vi "Database-Changeover.vi"(8 "error in":errorcluster, 10 "PLCchangeover":T2, 11 "Idx":i32) -> (0 "error out":errorcluster, 2 "PCchangeover":T1 {"TVH" format="%.3f"; "TVL" format="%.3f"; "TP" format="%.3f"})   [LabVIEW 2016]
doc: "Go to DB->WriteStationValues action\nReturn boolean flag to show if data was saved to DB successfully\n\nWabco 2017 All right reserved\nAuthor: maciej.szupienko@wabco-auto.com"
uses:
  Database.Action.ctl
  Drivers/PLC/LowLevel/PLC.DataBlock.PCchangeover.ctl
  Drivers/PLC/LowLevel/PLC.DataBlock.PLCchangeover.ctl
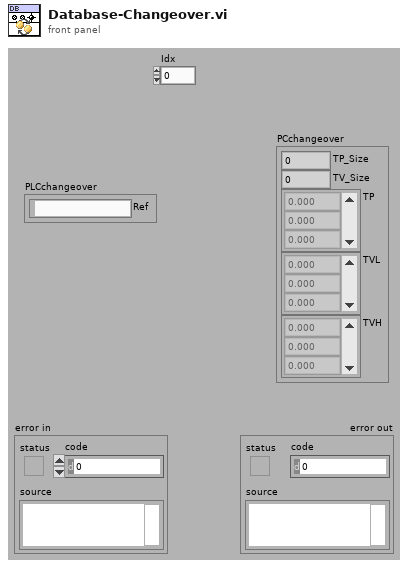
[diagram p1: front panel]
types:
  T1 = typedef "PLC.DataBlock.PCchangeover.ctl" = cluster{"TP_Size":u8, "TV_Size":u8, "TP":sgl[], "TVL":sgl[], "TVH":sgl[]}
  T2 = typedef "PLC.DataBlock.PLCchangeover.ctl" = cluster{"Ref":string}
  T3 = typedef "Database.Action.ctl" = enum32{"idle", "constructor", "destructor", "--- DB ---", "Setup", "Disconnect", "Connect", "GetAllStatuses"}
  T4 = typedef "Database.Data.Status.ctl" = cluster{"Run":bool, "Handle":i32, "ConnTS":timestamp, "DbTime":timestamp, "DbTimeOffset":dbl, "LastVariant":string, "LastSerial":string, "LastDataTS":timestamp, "LastStatus":i32}
  T5 = typedef "Cache.TestSteps.Fglb.TestData.ctl" = cluster{"Ref":string, "Desc":string, "P":T6, "PS":T7, "PP":T8[], "TS":cluster{"TS":T9, "TV":T10[], "TP":T11[]}[], "Units":T12[]}
  T6 = typedef "ProdaNG.Process.ctl" = cluster{"i_id":i32, "productionLineId":i32, "releaseId":i32, "contentId":string, "previewId":string, "mdReason":string, "mdUser":string, "mdTime":string, "description":string}
  T7 = typedef "ProdaNG.ProcessStep.ctl" = cluster{"i_id":i32, "processId":i32, "systemId":i32, "releaseId":i32, "processSequence":i32, "limitYellow":dbl, "limitRed":dbl, "mdReason":string, "mdUser":string, "mdTime":string, "filename":string, "transfer":string, "description":string}
  T8 = typedef "ProdaNG.ProcessStepParam.ctl" = cluster{"i_id":i32, "processStepId":i32, "unitId":i32, "contentId":string, "previewId":string, "value":dbl, "valueText":string, "paramSequence":i32, "history":i32, "mdReason":string, "mdUser":string, "mdTime":string, "description":string}
  T9 = typedef "ProdaNG.TestStep.ctl" = cluster{"i_id":i32, "processStepId":i32, "testSequence":i32, "testOrder":i32, "mdReason":string, "mdUser":string, "mdTime":string, "description":string}
  T10 = typedef "ProdaNG.TestValue.ctl" = cluster{"i_id":i32, "testStepId":i32, "releaseId":i32, "unitId":i32, "contentId":string, "previewId":string, "maximum":dbl, "minimum":dbl, "valueText":string, "testValueSequence":i32, "history":i32, "mdReason":string, "mdUser":string, "mdTime":string, "description":string}
  T11 = typedef "ProdaNG.TestStepParam.ctl" = cluster{"i_id":i32, "testStepId":i32, "unitId":i32, "contentId":string, "previewId":string, "value":dbl, "valueText":string, "paramSequence":i32, "history":i32, "mdReason":string, "mdUser":string, "mdTime":string, "description":string}
  T12 = typedef "ProdaNG.Unit.ctl" = cluster{"i_id":i32, "name":string, "mdReason":string, "mdUser":string, "mdTime":string, "description":string}
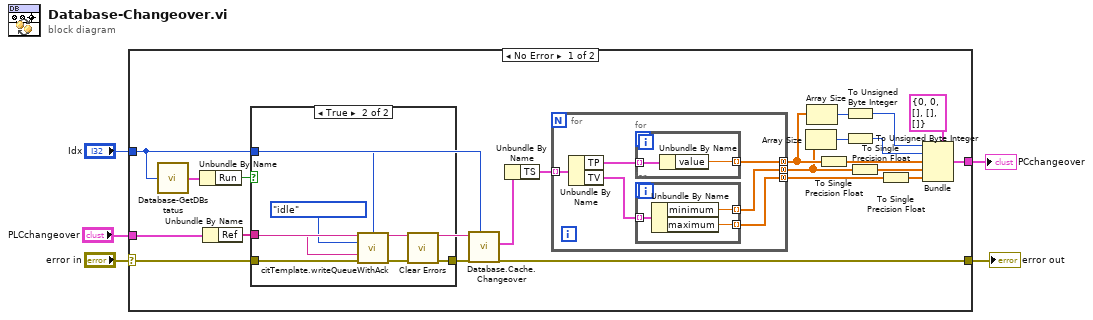
[diagram p0: block diagram]
diagram:
  n1 = case shown="No Error" "error in" {
    selector: "error in" -> [w27 w46]
    tunnel: [w24 w46] -> w4
    tunnel: "Idx" -> [w22 _]
    tunnel: "PLCchangeover" -> [w7 _]
    tunnel: [w11 _] -> w1
    frame No Error {
      n2 = call "Database-GetDBstatus.vi"("Idx"=w22) -> ("Status"=w26:T4)
      n3 = Unbundle By Name(w26) -> ("Run"=w25:bool)
      n4 = Unbundle By Name(w7) -> ("Ref"=w6:string)
      n5 = case shown="True" w25 {
        tunnel: w27 -> [w39 w45]
        tunnel: [w39 w42] -> w23
        tunnel: w22 -> [_ w44]
        tunnel: w6 -> [_ w41]
        frame False {
        }
        frame True {
          n6 = call "citTemplate.writeQueueWithAck.vi"("instance (0)"=w44, "event in"=Database.Action."idle" ("Action"), "(flatten) data in"=w41, "error in (no error)"=w45) -> ("error out"=w43:errorcluster)  [unwired: 9 in, 2 out]
          n7 = call <vilib>:"Clear Errors.vi"("error in (no error)"=w43) -> ("error out"=w42:errorcluster)  [unwired: 5 in, 1 out]
        }
      }
      n8 = call "Database.Cache.Changeover.vi"("Idx"=w22, "error in"=w23, "Ref"=w6) -> ("error out"=w24:errorcluster, "TS out"=w21:T5)  [unwired: 7 in]
      n9 = Unbundle By Name(w21) -> ("TS"=w20:cluster{"TS":T9, "TV":T10[], "TP":T11[]}[])
      n10 = for {
        tunnel: w20 -> [w33] mode=indexing
        tunnel: [w30] -> w15 mode=concatenating
        tunnel: [w29] -> w14 mode=concatenating
        tunnel: [w28] -> w19 mode=concatenating
        n11 = Unbundle By Name(w33) -> ("TP"=w32:T11[], "TV"=w31:T10[])
        n12 = for {
          tunnel: w32 -> [w38] mode=indexing
          tunnel: [w37] -> w30 mode=indexing
          n13 = Unbundle By Name(w38) -> ("value"=w37:dbl)
        }
        n14 = for {
          tunnel: w31 -> [w36] mode=indexing
          tunnel: [w35] -> w29 mode=indexing
          tunnel: [w34] -> w28 mode=indexing
          n15 = Unbundle By Name(w36) -> ("minimum"=w35:dbl, "maximum"=w34:dbl)
        }
      }
      n16 = Array Size(array=w14) -> (size(s)=w17:i32)
      n17 = Array Size(array=w15) -> (size(s)=w18:i32)
      n18 = To Single Precision Float(number=w15) -> (single precision float=w10:sgl[])
      n19 = To Unsigned Byte Integer(number=w18) -> (unsigned 8bit integer=w12:u8)
      n20 = To Unsigned Byte Integer(number=w17) -> (unsigned 8bit integer=w13:u8)
      n21 = To Single Precision Float(number=w14) -> (single precision float=w9:sgl[])
      n22 = To Single Precision Float(number=w19) -> (single precision float=w8:sgl[])
      n23 = Bundle(cluster=T1 {"TP_Size"=0, "TV_Size"=0, "TP"=[], "TVL"=[], "TVH"=[]} ("PCchangeover"), "TP_Size"=w12, "TV_Size"=w13, "TP"=w10, "TVL"=w9, "TVH"=w8) -> (w11:T1)
    }
    frame Error {
    }
  }
  "error out" <- w4
  "PCchangeover" <- w1
